vi "单个特征测试DMFCC.vi"() -> ()   [LabVIEW 2018]
panel:
  out "总用时（s）":dbl
  out "结束时间（ms）":u32
  out "开始时间（ms）":u32
  out "说话人序号":i32
  out "所有距离":dbl[](array[numeric])
  out "下阈值":dbl
  out "上阈值":dbl
  out "识别完成":bool
  out "训练完成":bool
  out "特征参数":dbl[][](graph)
  out "加窗分帧后":dbl[][](graph)
  out "滤波后":dbl[][](graph)
  out "待识别语音":dbl[][](graph)
  out "提示框":string
  in  "说话人 6":path=path "D:/Desktop/audio/train/胡楠.lvm"
  in  "说话人 5":path=path "D:/Desktop/audio/train/1234.lvm"
  in  "说话人 4":path=path "D:/Desktop/audio/train/anjiale1.lvm"
  in  "说话人 3":path=path "D:/Desktop/audio/train/赵霞.lvm"
  in  "说话人 2":path=path "D:/Desktop/audio/train/叶雪花.lvm"
  in  "说话人 1":path=path "D:/Desktop/audio/train/zhuqiseng1.lvm"
  out "确定的人":string
  out "距离":dbl format="%.2f"
  in  "语音识别":bool
  in  "语音训练":bool
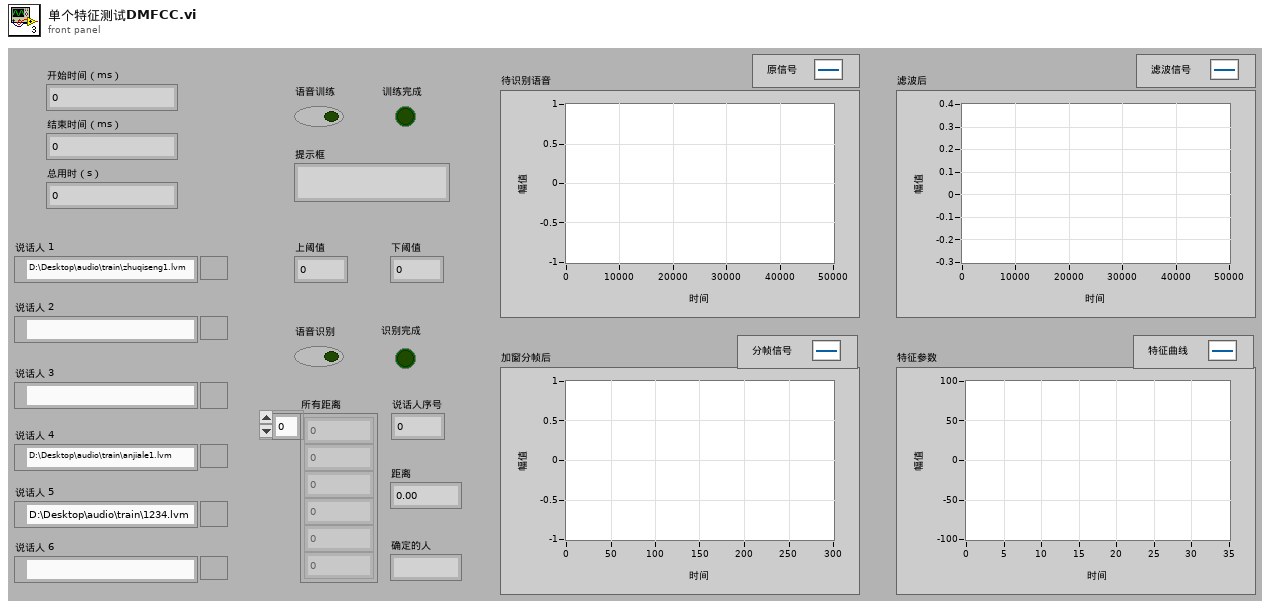
[diagram p1: front panel]
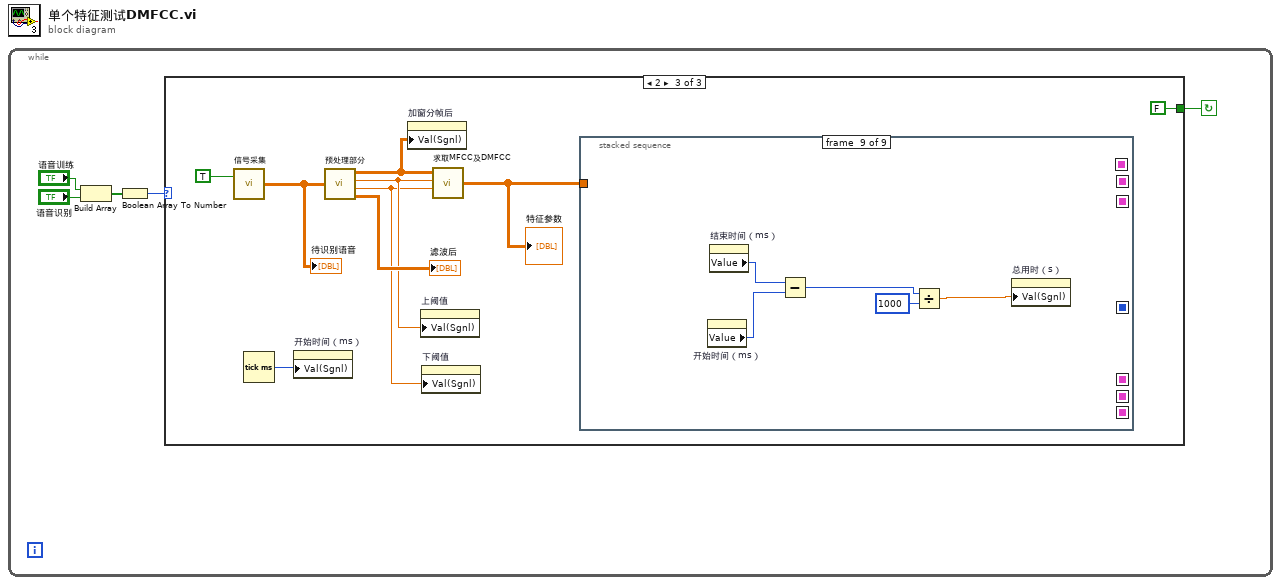
[diagram p0: block diagram]
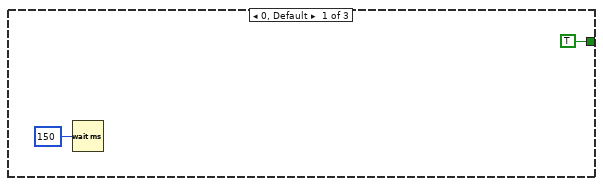
[diagram p2: hidden frame]
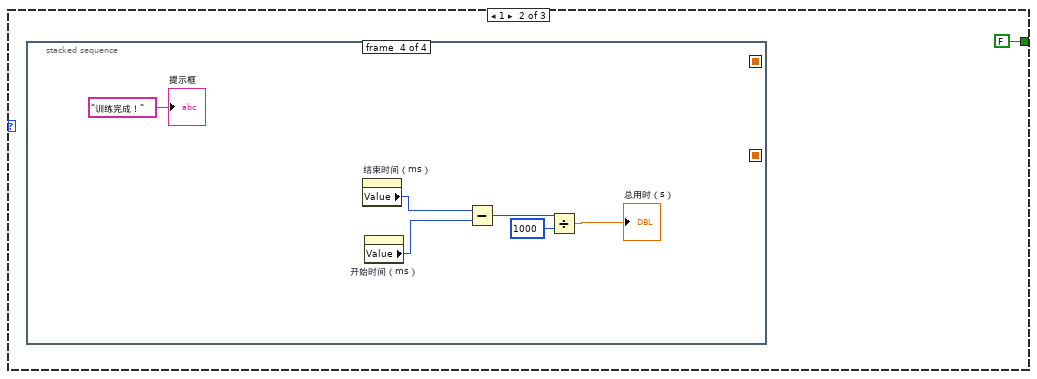
[diagram p3: hidden frame]
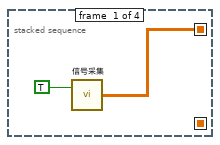
[diagram p4: hidden frame]
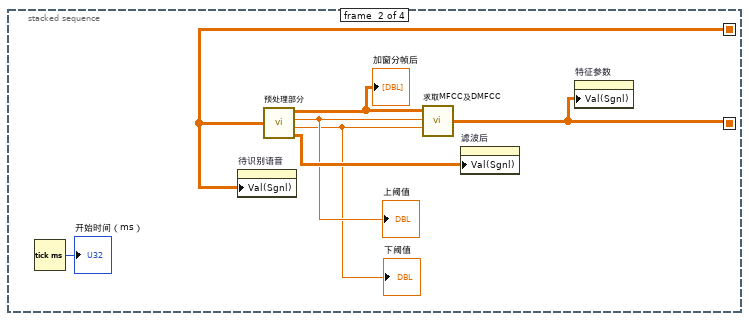
[diagram p5: hidden frame]
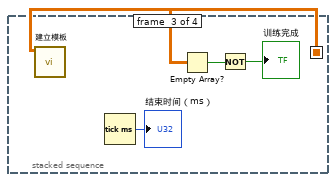
[diagram p6: hidden frame]
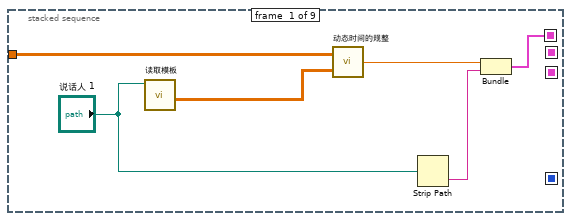
[diagram p7: hidden frame]
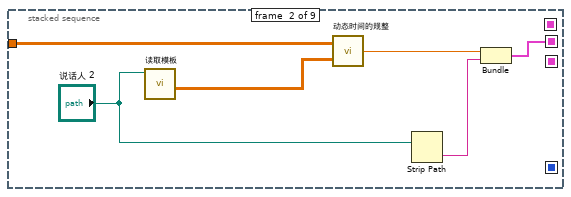
[diagram p8: hidden frame]
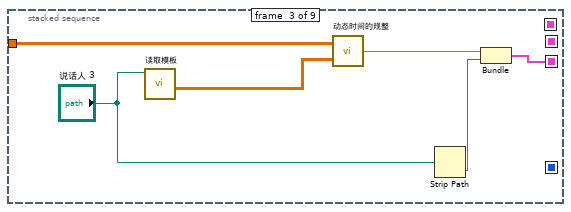
[diagram p9: hidden frame]
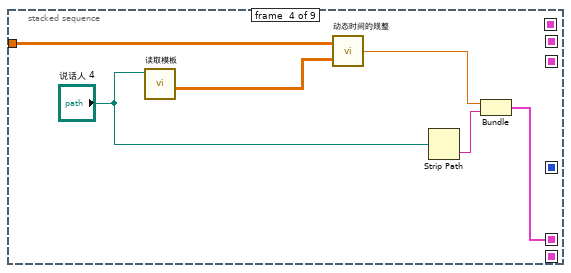
[diagram p10: hidden frame]
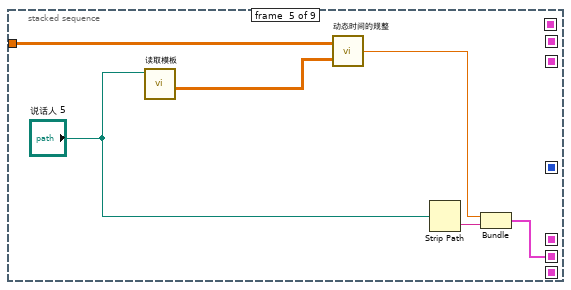
[diagram p11: hidden frame]
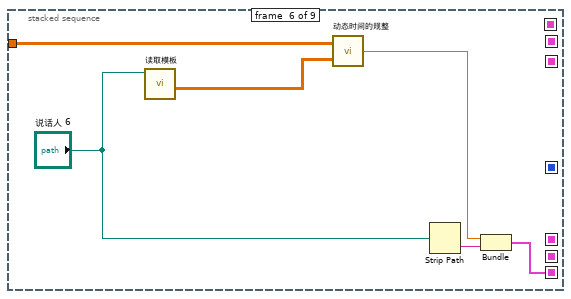
[diagram p12: hidden frame]
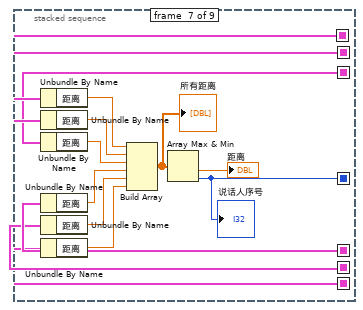
[diagram p13: hidden frame]
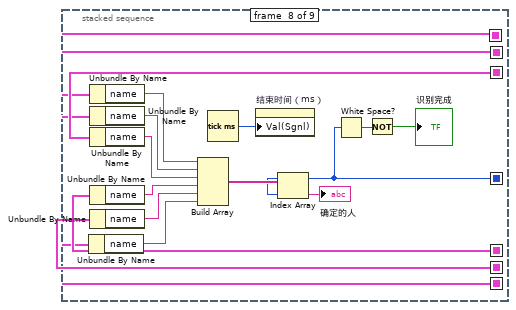
[diagram p14: hidden frame]
diagram:
  n1 = while {
    stop <- w1 continue-if-true
    n2 = Build Array("语音训练", "语音识别") -> (w3:bool[])
    n3 = Boolean Array To Number(Boolean array=w3) -> (number=w2:u32)
    n4 = case shown="2" w2 {
      tunnel: [TRUE FALSE FALSE] -> w1
      frame 0, Default {
        n5 = Wait (ms)(milliseconds to wait=u32 150) -> ()  [unwired: 1 out]
      }
      frame 1 {
        n6 = stacked-sequence {
          seq-local: [_ w13 _ _] -> [_ _ w20 _]
          seq-local: [w9 _ _ _] -> [_ w11 _ _]
          frame #0 {
            n7 = call "信号采集.vi"("Boolean"=TRUE) -> ("mono 16-bit"=w9:dbl[][])  [unwired: 1 in]
          }
          frame #1 {
            n8 = Tick Count (ms)() -> (millisecond timer value=→"开始时间（ms）":u32)
            n9 = property on="待识别语音" class="WFGraph (严格)"("Val(Sgnl)"=w11) -> ()  [unwired: 2 in, 2 out]
            n10 = call "预处理部分.vi"("mono 16-bit"=w11) -> ("y"=w16:dbl[][], "s1"=w15:dbl, "s2"=w14:dbl, "波形图 2"=w17:dbl[][])
            "加窗分帧后" <- w16
            "上阈值" <- w15
            "下阈值" <- w14
            n11 = call "求取MFCC及DMFCC.vi"("s2"=w14, "s1"=w15, "xx"=w16) -> ("MFCC DTM"=w13:dbl[][])
            n12 = property on="滤波后" class="WFGraph (严格)"("Val(Sgnl)"=w17) -> ()  [unwired: 2 in, 2 out]
            n13 = property on="特征参数" class="WFGraph (严格)"("Val(Sgnl)"=w13) -> ()  [unwired: 2 in, 2 out]
          }
          frame #2 {
            n14 = call "建立模板.vi"("输入MFCC"=w20) -> ()  [unwired: 11 in]
            n15 = Tick Count (ms)() -> (millisecond timer value=→"结束时间（ms）":u32)
            n16 = Empty Array?(array=w20) -> (empty?=w21:bool)
            n17 = Not(x=w21) -> (.not. x?=→"训练完成":bool)
          }
          frame #3 {
            n18 = property on="结束时间（ms）" class="DigNum (严格)"() -> ("Value"=w23:u32)  [unwired: 2 in, 2 out]
            n19 = property on="开始时间（ms）" class="DigNum (严格)"() -> ("Value"=w22:u32)  [unwired: 2 in, 2 out]
            n20 = Subtract(x=w23, y=w22) -> (x-y=w26:u32)
            n21 = Divide(x=w26, y=u32 1000) -> (x/y=→"总用时（s）":dbl)
            "提示框" <- "训练完成！"
          }
        }
      }
      frame 2 {
        n22 = call "信号采集.vi"("Boolean"=TRUE) -> ("mono 16-bit"=w34:dbl[][])  [unwired: 1 in]
        "待识别语音" <- w34
        n23 = Tick Count (ms)() -> (millisecond timer value=w28:u32)
        n24 = property on="开始时间（ms）" class="DigNum (严格)"("Val(Sgnl)"=w28) -> ()  [unwired: 2 in, 2 out]
        n25 = call "预处理部分.vi"("mono 16-bit"=w34) -> ("y"=w32:dbl[][], "s1"=w30:dbl, "s2"=w29:dbl, "波形图 2"=→"滤波后":dbl[][])
        n26 = property on="加窗分帧后" class="WFGraph (严格)"("Val(Sgnl)"=w32) -> ()  [unwired: 2 in, 2 out]
        n27 = property on="上阈值" class="DigNum (严格)"("Val(Sgnl)"=w30) -> ()  [unwired: 2 in, 2 out]
        n28 = property on="下阈值" class="DigNum (严格)"("Val(Sgnl)"=w29) -> ()  [unwired: 2 in, 2 out]
        n29 = call "求取MFCC及DMFCC.vi"("s2"=w29, "s1"=w30, "xx"=w32) -> ("MFCC DTM"=w31:dbl[][])
        "特征参数" <- w31
        n30 = stacked-sequence {
          seq-local: [_ _ _ _ _ _ w73 _ _] -> [_ _ _ _ _ _ _ w91 _]
          seq-local: [w38 _ _ _ _ _ _ _ _] -> [_ _ _ _ _ _ w87 w96 _]
          seq-local: [_ w44 _ _ _ _ _ _ _] -> [_ _ _ _ _ _ w86 w97 _]
          seq-local: [_ _ w50 _ _ _ _ _ _] -> [_ _ _ _ _ _ w85 w98 _]
          seq-local: [_ _ _ w56 _ _ _ _ _] -> [_ _ _ _ _ _ w84 w95 _]
          seq-local: [_ _ _ _ w62 _ _ _ _] -> [_ _ _ _ _ _ w83 w94 _]
          seq-local: [_ _ _ _ _ w68 _ _ _] -> [_ _ _ _ _ _ w82 w93 _]
          tunnel: w31 -> [w42 w48 w53 w59 w65 w71 _ _ _]
          frame #0 {
            n31 = call "读取模板.vi"("Filename"="说话人 1") -> ("模板特征参数 2"=w41:dbl[][])  [unwired: 10 in]
            n32 = call "动态时间的规整.vi"("参考模板特征"=w41, "²âÊÔÄ£°åÌØÕ÷Å"=w42) -> ("距离"=w40:dbl)
            n33 = Strip Path(path="说话人 1") -> (name=w39:string)  [unwired: 1 out]
            n34 = Bundle("距离"=w40, "name"=w39) -> (w38:cluster{"距离":dbl, "name":string})  [unwired: 1 in]
          }
          frame #1 {
            n35 = call "读取模板.vi"("Filename"="说话人 2") -> ("模板特征参数 2"=w47:dbl[][])  [unwired: 10 in]
            n36 = call "动态时间的规整.vi"("参考模板特征"=w47, "²âÊÔÄ£°åÌØÕ÷Å"=w48) -> ("距离"=w46:dbl)
            n37 = Strip Path(path="说话人 2") -> (name=w45:string)  [unwired: 1 out]
            n38 = Bundle("距离"=w46, "name"=w45) -> (w44:cluster{"距离":dbl, "name":string})  [unwired: 1 in]
          }
          frame #2 {
            n39 = call "读取模板.vi"("Filename"="说话人 3") -> ("模板特征参数 2"=w54:dbl[][])  [unwired: 10 in]
            n40 = call "动态时间的规整.vi"("参考模板特征"=w54, "²âÊÔÄ£°åÌØÕ÷Å"=w53) -> ("距离"=w52:dbl)
            n41 = Strip Path(path="说话人 3") -> (name=w51:string)  [unwired: 1 out]
            n42 = Bundle("距离"=w52, "name"=w51) -> (w50:cluster{"距离":dbl, "name":string})  [unwired: 1 in]
          }
          frame #3 {
            n43 = call "读取模板.vi"("Filename"="说话人 4") -> ("模板特征参数 2"=w60:dbl[][])  [unwired: 10 in]
            n44 = call "动态时间的规整.vi"("参考模板特征"=w60, "²âÊÔÄ£°åÌØÕ÷Å"=w59) -> ("距离"=w58:dbl)
            n45 = Strip Path(path="说话人 4") -> (name=w57:string)  [unwired: 1 out]
            n46 = Bundle("距离"=w58, "name"=w57) -> (w56:cluster{"距离":dbl, "name":string})  [unwired: 1 in]
          }
          frame #4 {
            n47 = call "读取模板.vi"("Filename"="说话人 5") -> ("模板特征参数 2"=w66:dbl[][])  [unwired: 10 in]
            n48 = call "动态时间的规整.vi"("参考模板特征"=w66, "²âÊÔÄ£°åÌØÕ÷Å"=w65) -> ("距离"=w64:dbl)
            n49 = Strip Path(path="说话人 5") -> (name=w63:string)  [unwired: 1 out]
            n50 = Bundle("距离"=w64, "name"=w63) -> (w62:cluster{"距离":dbl, "name":string})  [unwired: 1 in]
          }
          frame #5 {
            n51 = call "读取模板.vi"("Filename"="说话人 6") -> ("模板特征参数 2"=w72:dbl[][])  [unwired: 10 in]
            n52 = call "动态时间的规整.vi"("参考模板特征"=w72, "²âÊÔÄ£°åÌØÕ÷Å"=w71) -> ("距离"=w70:dbl)
            n53 = Strip Path(path="说话人 6") -> (name=w69:string)  [unwired: 1 out]
            n54 = Bundle("距离"=w70, "name"=w69) -> (w68:cluster{"距离":dbl, "name":string})  [unwired: 1 in]
          }
          frame #6 {
            n55 = Unbundle By Name(w87) -> ("距离"=w81:dbl)
            n56 = Unbundle By Name(w86) -> ("距离"=w80:dbl)
            n57 = Unbundle By Name(w85) -> ("距离"=w79:dbl)
            n58 = Unbundle By Name(w84) -> ("距离"=w78:dbl)
            n59 = Unbundle By Name(w83) -> ("距离"=w77:dbl)
            n60 = Unbundle By Name(w82) -> ("距离"=w76:dbl)
            n61 = Build Array(w81, w80, w79, w78, w77, w76) -> (w74:dbl[])
            "所有距离" <- w74
            n62 = Array Max & Min(array=w74) -> (min value=→"距离":dbl, min index (indices)=w73:i32)  [unwired: 2 out]
            "说话人序号" <- w73
          }
          frame #7 {
            n63 = Unbundle By Name(w93) -> ("name"=w99:string)
            n64 = Unbundle By Name(w96) -> ("name"=w104:string)
            n65 = Unbundle By Name(w97) -> ("name"=w103:string)
            n66 = Unbundle By Name(w98) -> ("name"=w102:string)
            n67 = Unbundle By Name(w95) -> ("name"=w101:string)
            n68 = Unbundle By Name(w94) -> ("name"=w100:string)
            n69 = Build Array(w104, w103, w102, w101, w100, w99) -> (w105:string[])
            n70 = Tick Count (ms)() -> (millisecond timer value=w88:u32)
            n71 = property on="结束时间（ms）" class="DigNum (严格)"("Val(Sgnl)"=w88) -> ()  [unwired: 2 in, 2 out]
            n72 = Index Array(array=w105, index=w91) -> (element=→"确定的人":string)
            n73 = White Space?(1:w91) -> (0:w90:bool)
            n74 = Not(x=w90) -> (.not. x?=→"识别完成":bool)
          }
          frame #8 {
            n75 = property on="开始时间（ms）" class="DigNum (严格)"() -> ("Value"=w108:u32)  [unwired: 2 in, 2 out]
            n76 = property on="结束时间（ms）" class="DigNum (严格)"() -> ("Value"=w109:u32)  [unwired: 2 in, 2 out]
            n77 = Subtract(x=w109, y=w108) -> (x-y=w106:u32)
            n78 = Divide(x=w106, y=u32 1000) -> (x/y=w107:dbl)
            n79 = property on="总用时（s）" class="DigNum (严格)"("Val(Sgnl)"=w107) -> ()  [unwired: 2 in, 2 out]
          }
        }
      }
    }
  }
